vi "读取Excel至多列列表框.vi"(8 "error in (no error)":errorcluster caption="错误输入（无错误）", 11 "Excel表格路径":path caption="模板（空）") -> (0 "error out":errorcluster, 1 "混响数值":string[][](array[string]), 2 "列首":string[](array[string]), 3 "行首":string[](array[string]))   [LabVIEW 2020]
uses:
  <vilib>/Utility/NIReport.llb/Report Type.ctl
  <vilib>/addons/_office/excel.llb/Excel Get Data ([str]).vi
  <vilib>/addons/_office/NI_ReportGenerationToolkit.lvlib
  <vilib>/Utility/NIReport.llb/NI_report.lvclass
  <vilib>/Utility/NIReport.llb/NI_ReportGenerationCore.lvlib
  <vilib>/Utility/NIReport.llb/Excel/NI_Excel.lvclass
panel:
  out "所有数据":string[][](array[string])
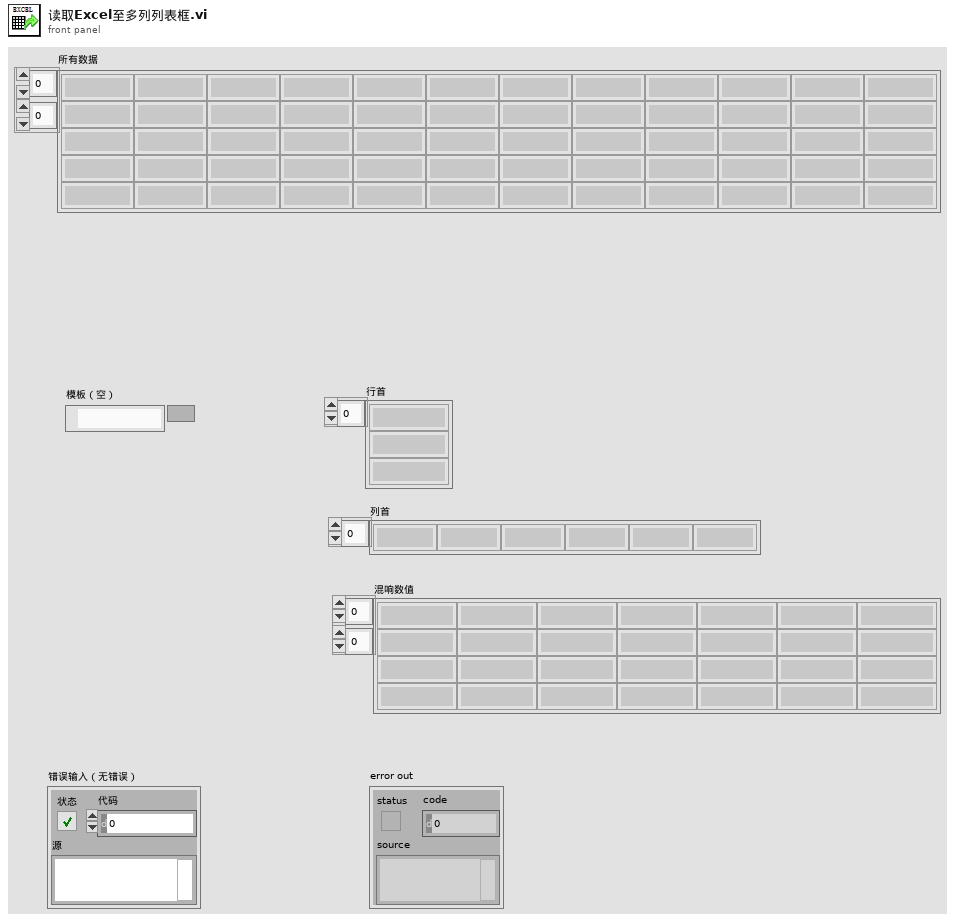
[diagram p1: front panel]
types:
  T1 = typedef "NI_ReportGenerationCore.lvlib/Report Type.ctl" = enum16{"HTML", "Word", "Excel"}
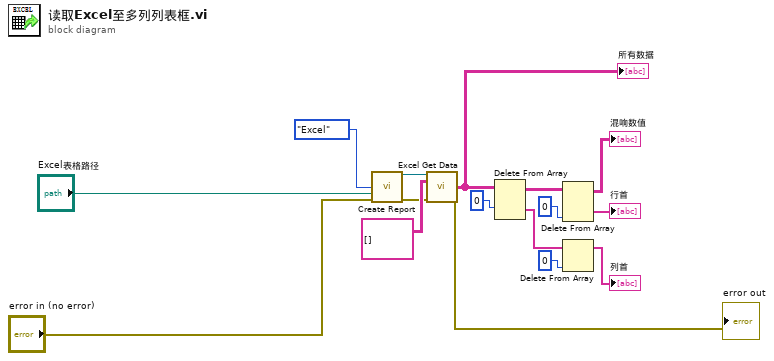
[diagram p0: block diagram]
diagram:
  n1 = call <vilib>:"Create Report.vi"("report type"=Report_Type."Excel", "template (empty)"="Excel表格路径", "error in (no error)"="error in (no error)") -> ("report out"=w16:refnum<class "NI_report.lvclass">, "error out"=w1:errorcluster)  [unwired: 11 in]
  n2 = call-poly <vilib>:"Excel Get Data.vi"("report in"=w16, "data type"=string[][] [], "error in (no error)"=w1) -> ("data"=w10:string[][], "error out"=→"error out":errorcluster)  [unwired: 10 in, 1 out]
  "所有数据" <- w10
  n3 = Delete From Array(array=w10, index (row)=0 ("索引")) -> (deleted portion=w7:string[], array with subset deleted=w12:string[][])  [unwired: 2 in]
  n4 = Delete From Array(array=w12, index (col)=0 ("禁用的索引 (列)")) -> (deleted portion=→"行首":string[], array with subset deleted=→"混响数值":string[][])  [unwired: 2 in]
  n5 = Delete From Array(array=w7, index=0 ("索引")) -> (array with subset deleted=→"列首":string[])  [unwired: 1 in, 1 out]
